vi "Write X.vi"(8 "error in (no error)":errorcluster, 10 "X":dbl, 11 "JumpAbs in":refnum<class "JumpRel.lvclass">) -> (0 "error out":errorcluster, 3 "JumpAbs out":refnum<class "JumpRel.lvclass">)   [LabVIEW 2013, in "HardwareCharacterization.lvlib" / "JumpRel.lvclass"]
uses:
  JumpRel.lvclass
  JumpRel.lvclass/JumpRel.ctl
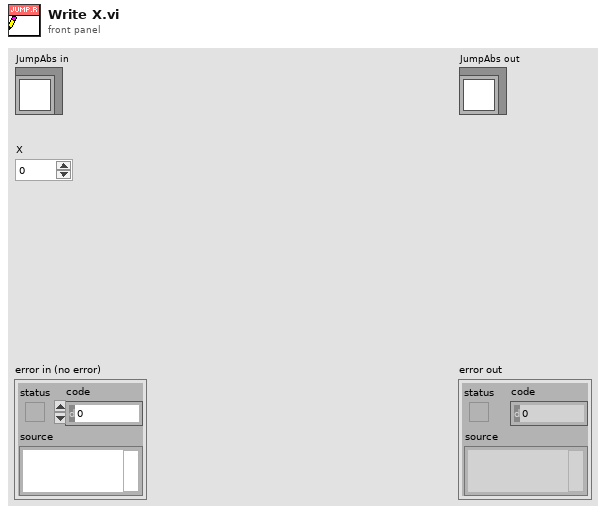
[diagram p1: front panel]
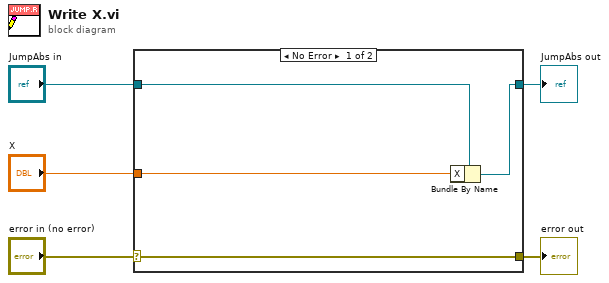
[diagram p0: block diagram]
diagram:
  n1 = case shown="No Error" "error in (no error)" {
    selector: "error in (no error)" -> [w9 w10]
    tunnel: [w9 w10] -> w4
    tunnel: [w7 w11] -> w2
    tunnel: "JumpAbs in" -> [w8 w11]
    tunnel: "X" -> [w6 _]
    frame No Error {
      n2 = Bundle By Name(cluster=w8, "X"=w6) -> (w7:refnum<class "JumpRel.lvclass">)
    }
    frame Error {
    }
  }
  "error out" <- w4
  "JumpAbs out" <- w2
